vi "Add Key Value To Profile.vi"(8 "error in (no error)":errorcluster, 9 "Value":string, 10 "Key":string, 11 "Output Actor Hardware in":refnum<class "Output Actor Hardware.lvclass">) -> (0 "error out":errorcluster, 3 "Output Actor Hardware out":refnum<class "Output Actor Hardware.lvclass">)   [LabVIEW 2015, in "Output Actor Hardware.lvclass"]
uses:
  Output Actor Hardware.lvclass
  Output Actor Hardware.lvclass/Output Actor Hardware.ctl
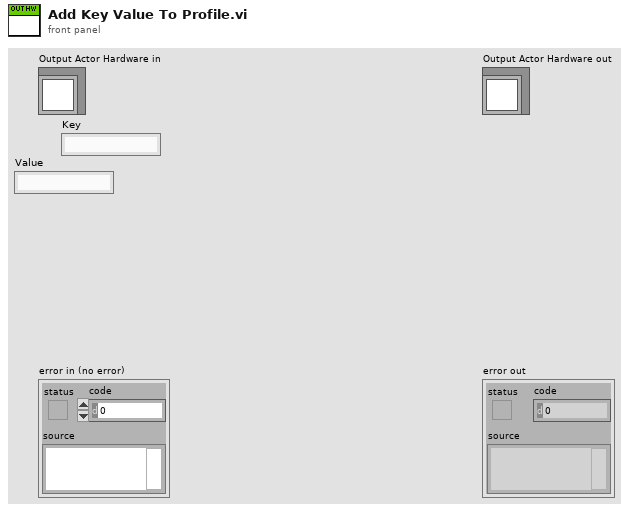
[diagram p1: front panel]
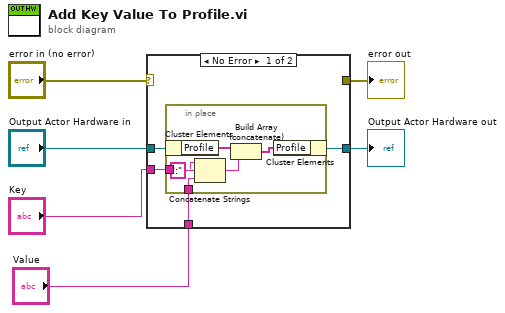
[diagram p0: block diagram]
diagram:
  n1 = case shown="No Error" "error in (no error)" {
    selector: "error in (no error)" -> [_ w18]
    tunnel: [_ w18] -> w5
    tunnel: [w9 w17] -> w3
    tunnel: "Output Actor Hardware in" -> [w10 w17]
    tunnel: "Key" -> [w8 _]
    tunnel: "Value" -> [w7 _]
    frame No Error {
      n2 = in-place {
        in-place-border: w8 -> [w13]
        in-place-border: w7 -> [w12]
        n3 = in-place-cluster #1(w10) -> ("Profile"=w16:string[])
        n4 = Concatenate Strings(w13, ":" ("string"), w12) -> (w11:string)
        n5 = Build Array (concatenate)(w16, w11) -> (w15:string[])
        n6 = in-place-cluster #1("Profile"=w15) -> (w9:refnum<class "Output Actor Hardware.lvclass">)
      }
    }
    frame Error {
    }
  }
  "error out" <- w5
  "Output Actor Hardware out" <- w3
